vi "Colorbar.vi"(5 "Tick Labels":string[](array[string]), 7 "Ticks":dbl[](array[numeric]), 8 "error in (no error)":errorcluster, 10 "Label":string, 11 "Plot ID":T1 format="%x") -> (0 "error out":errorcluster, 3 "Plot ID Out":T1 format="%x")   [LabVIEW 2013, in "Advanced Plotting Toolkit.lvlib"]
doc: "Add a colorbar to the right of the existing axes. The colormap and range values are taken from the last colormapped object plotted.\n\nIf no colormapped object has been plotted, has no effect."
uses:
  Advanced Plotting Toolkit.lvlib
  typedefs/PlotID.ctl
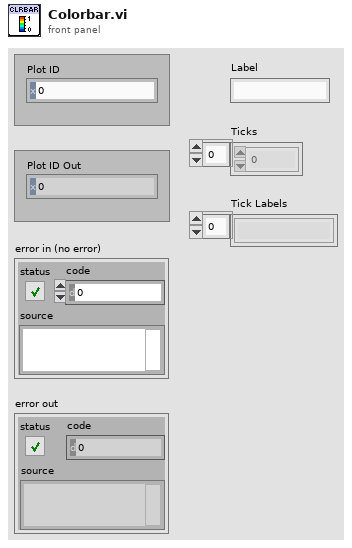
[diagram p1: front panel]
types:
  T1 = typedef "Advanced Plotting Toolkit.lvlib/PlotID.ctl" = i32
  T2 = typedef "Advanced Plotting Toolkit.lvlib/KeyValue.ctl" = cluster{"Key":string, "Value":string}
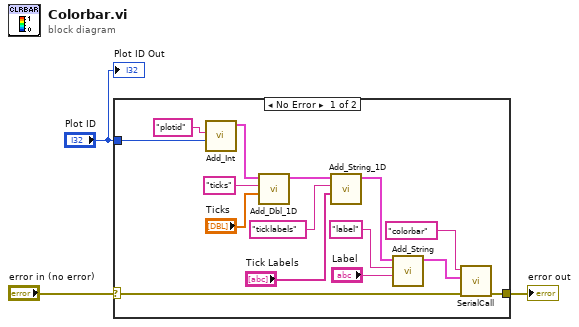
[diagram p0: block diagram]
diagram:
  n1 = case shown="No Error" "error in (no error)" {
    selector: "error in (no error)" -> [w17 w19]
    tunnel: "Plot ID" -> [w18 _]
    tunnel: [w16 w19] -> w1
    frame No Error {
      n2 = call "Add_Int.vi"("Value"=w18, "Key"="plotid") -> ("Keyword Array Out"=w13:T2[])  [unwired: 9 in]
      n3 = call "Add_Dbl_1D.vi"("Value"="Ticks", "Key"="ticks", "Keyword Array"=w13) -> ("Keyword Array Out"=w10:T2[])  [unwired: 8 in]
      n4 = call "Add_String_1D.vi"("Value"="Tick Labels", "Key"="ticklabels", "Keyword Array"=w10) -> ("Keyword Array Out"=w7:T2[])  [unwired: 8 in]
      n5 = call "Add_String.vi"("Value"="Label", "Key"="label", "Keyword Array"=w7) -> ("Keyword Array Out"=w4:T2[])  [unwired: 8 in]
      n6 = call "SerialCall.vi"("error in (no error)"=w17, "data"=w4, "Resource"="colorbar") -> ("error out"=w16:errorcluster)  [unwired: 7 in, 1 out]
    }
    frame Error {
    }
  }
  "error out" <- w1
  "Plot ID Out" <- "Plot ID"
